vi "Nonlinear Calibration Test v3.vi"() -> ()   [LabVIEW 2009]
doc: "This example illustrates the use of a calibration grid to calibrate and correct an image for nonlinear distortion and accurate shape measurements.\n\nThis example loads the image of a calibration grid used to calibrate the system, learns the grid, then loads an image of parts acquired using the same setup. The example then corrects the image in two ways. The first method corrects the entire image and then measures the area of the coins. The second method corrects only the area of the coins and displays the difference in processing time."
uses:
  <vilib>/vision/NI_Vision_Development_Module.lvlib
panel:
  out "Bottom Image":T1(plugin-control) caption="Coins Image"
  out "Top Image":T1(plugin-control) caption="Calibration Template"
  out "time (ms) to correct":u32
  out "time (ms) to correct":u32
  in  "Load Image of Parts":bool
  in  "Return":bool
  in  "Measure Parts":bool
  in  "Learn Calibration":bool
  in  "Load Calibration Template":bool
  # "1. Loads the image of a calibration grid that is used to calibrate the system."
  # "2. Learn the calibration grid. Note that this process is computation intensive and needs a fair amount of time to complete."
  # "3. Load Image of Parts acquired using the same setup."
  # "4. Correct the image and measure areas of the objects in the image."
  # "This step takes measurements in two ways.  The first calculation corrects \nthe entire image, and then takes the measurements.  The second calculation only corrects the coins, and then takes the measurements."
  # "time (ms) to correct entire image, threshold and calculate measurements"
  # "time (ms) to threshold, correct just coins, and then take measurements"
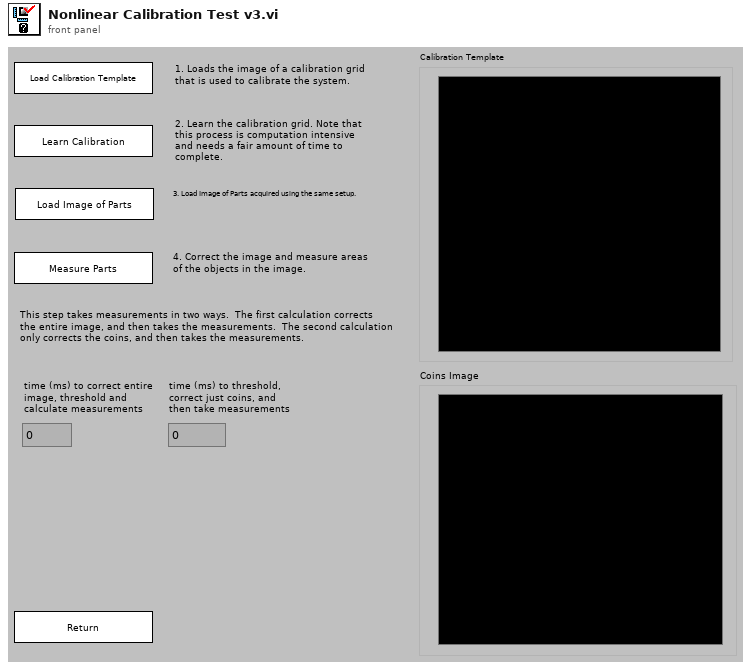
[diagram p1: front panel]
types:
  T1 = typedef "IMAQ Image.ctl" = refnum<image>
  T2 = cluster{"X Step":sgl, "Y Step":sgl, "Unit":u32, "Threshold Range":cluster{"Lower value":sgl, "Upper value":sgl}}
  T3 = cluster{"Distortion":u32, "Corrected Image Scaling":u32, "Corrected Image Learn ROI":u32, "Learn Error Map?":bool, "Learn Correction Table?":bool}
  T4 = typedef "Particle Parameters" = i32
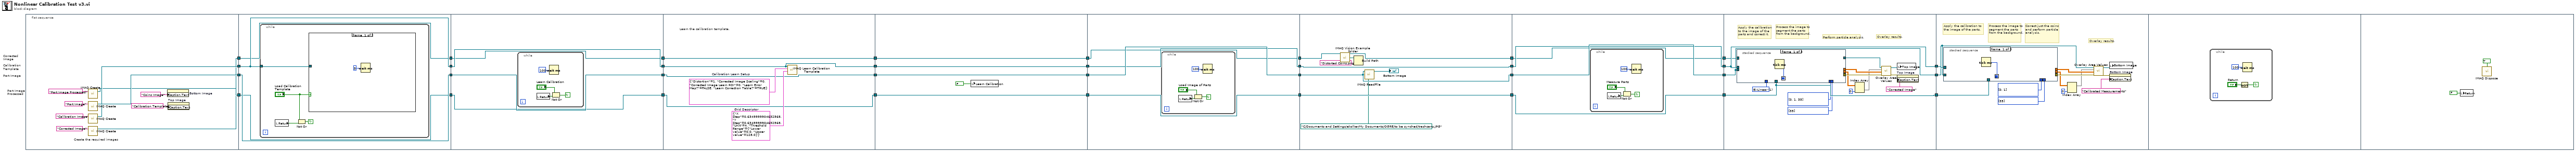
[diagram p0: block diagram]
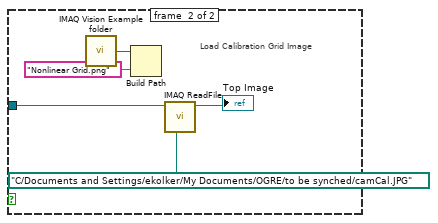
[diagram p2: hidden frame]
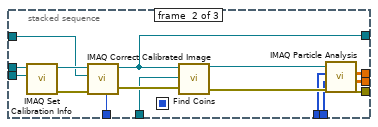
[diagram p3: hidden frame]
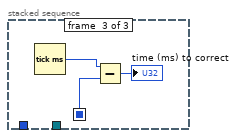
[diagram p4: hidden frame]
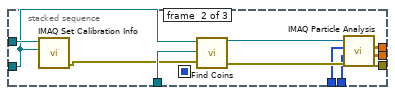
[diagram p5: hidden frame]
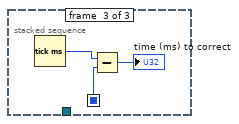
[diagram p6: hidden frame]
diagram:
  # "Corrected\nImage"
  # "Part Image Processed"
  # "Calibration Template"
  # "Part Image"
  n1 = flat-sequence {
    tunnel: [w44] -> w35
    tunnel: [w42] -> w34
    tunnel: [w40] -> w33
    tunnel: [w38] -> w32
    tunnel: w35 -> [w48]
    tunnel: [w48] -> w31
    tunnel: w34 -> [w49]
    tunnel: [w49] -> w30
    tunnel: w33 -> [w47]
    tunnel: [w47] -> w29
    tunnel: w32 -> [w46]
    tunnel: [w46] -> w28
    tunnel: w31 -> [w63]
    tunnel: [w63] -> w27
    tunnel: w30 -> [w62]
    tunnel: [w62] -> w26
    tunnel: w29 -> [w61]
    tunnel: [w61] -> w25
    tunnel: w28 -> [w60]
    tunnel: [w60] -> w24
    tunnel: w27 -> [w70]
    tunnel: [w70] -> w23
    tunnel: w26 -> [w73]
    tunnel: [w73] -> w22
    tunnel: w25 -> [w69]
    tunnel: [w69] -> w21
    tunnel: w24 -> [w68]
    tunnel: [w68] -> w20
    tunnel: w23 -> [w77]
    tunnel: [w77] -> w19
    tunnel: w22 -> [w76]
    tunnel: [w76] -> w18
    tunnel: w21 -> [w75]
    tunnel: [w75] -> w17
    tunnel: w20 -> [w74]
    tunnel: [w74] -> w16
    tunnel: w19 -> [w82]
    tunnel: [w82] -> w15
    tunnel: w18 -> [w81]
    tunnel: [w81] -> w14
    tunnel: w17 -> [w80]
    tunnel: [w80] -> w13
    tunnel: w16 -> [w79]
    tunnel: [w79] -> w12
    tunnel: w15 -> [w94]
    tunnel: [w94] -> w11
    tunnel: w14 -> [w90]
    tunnel: [w90] -> w10
    tunnel: w13 -> [w89]
    tunnel: [w89] -> w9
    tunnel: w12 -> [w88]
    tunnel: [w88] -> w8
    tunnel: w11 -> [w98]
    tunnel: [w98] -> w7
    tunnel: w10 -> [w97]
    tunnel: [w97] -> w6
    tunnel: w9 -> [w96]
    tunnel: [w96] -> w5
    tunnel: w8 -> [w95]
    tunnel: [w95] -> w4
    tunnel: w7 -> [w117]
    tunnel: [w117] -> w3
    tunnel: w6 -> [w118]
    tunnel: [w118] -> w2
    tunnel: w5 -> [w116]
    tunnel: [w116] -> w1
    tunnel: w4 -> [w114]
    tunnel: w3 -> [w144]
    tunnel: w2 -> [w151]
    tunnel: w1 -> [w150]
    frame #0 {
      # "Create the required images"
      n2 = call "IMAQ Create"("Image Name"="Calibration Image") -> ("New Image"=w42:T1)  [unwired: 3 in, 2 out]
      n3 = call "IMAQ Create"("Image Name"="Corrected Image") -> ("New Image"=w38:T1)  [unwired: 3 in, 2 out]
      n4 = call "IMAQ Create"("Image Name"="Part Image Processed") -> ("New Image"=w40:T1)  [unwired: 3 in, 2 out]
      n5 = call "IMAQ Create"("Image Name"="Part Image") -> ("New Image"=w44:T1)  [unwired: 3 in, 2 out]
      n6 = property on="Bottom Image" class="ImageControl"("Caption.Text"="Coins Image" ("Title")) -> ()  [unwired: 2 in, 2 out]
      n7 = property on="Top Image" class="ImageControl"("Caption.Text"="Calibration Template" ("Title")) -> ()  [unwired: 2 in, 2 out]
    }
    frame #1 {
      n8 = while {
        tunnel: w49 -> [w53]
        stop <- w51 continue-if-true
        n9 = local read "Return"() -> (w50:bool)
        n10 = Not Or(1:w50, 2:"Load Calibration Template") -> (0:w51:bool)
        n11 = case shown="True" "Load Calibration Template" {
          tunnel: w53 -> [_ w59]
          frame #0 {
            n12 = Wait (ms)(milliseconds to wait=u32 5) -> ()  [unwired: 1 out]
          }
          frame #1 {
            # "Load Calibration Grid Image"
            n13 = call "IMAQ Vision Example folder.vi"() -> ("Example Image Path"=w58:path)  [unwired: 1 out]
            n14 = Build Path(base path=w58, name or relative path="Nonlinear Grid.png") -> ()  [unwired: 1 out]
            n15 = call "IMAQ ReadFile"("File Path"=path "C:/Documents and Settings/ekolker/My Documents/OGRE/to be synched/camCal.JPG", "Image"=w59) -> ("Image Out"=→"Top Image":T1)  [unwired: 3 in, 6 out]
          }
        }
      }
    }
    frame #2 {
      # "Wait for Learn Calibration Button press"
      n16 = while {
        stop <- w65 continue-if-true
        n17 = local read "Return"() -> (w66:bool)
        n18 = Wait (ms)(milliseconds to wait=u32 100) -> ()  [unwired: 1 out]
        n19 = Not Or(1:w66, 2:"Learn Calibration") -> (0:w65:bool)
      }
    }
    frame #3 {
      w71 = T2 {"X Step"=0.635, "Y Step"=0.635, "Unit"=4, "Threshold Range"={"Lower value"=0.0, "Upper value"=128.0}}  # Grid Descriptor
      w72 = T3 {"Distortion"=1, "Corrected Image Scaling"=0, "Corrected Image Learn ROI"=0, "Learn Error Map?"=FALSE, "Learn Correction Table?"=TRUE}  # Calibration Learn Setup
      # "Learn the calibration template."
      n20 = call "IMAQ Learn Calibration Template"("Grid Descriptor"=w71, "Calibration Learn Setup"=w72, "Image"=w73) -> ()  [unwired: 4 in, 5 out]
    }
    frame #4 {
      n21 = local write "Learn Calibration"(FALSE ("Learn Calibration")) -> ()
    }
    frame #5 {
      n22 = while {
        stop <- w84 continue-if-true
        n23 = local read "Return"() -> (w85:bool)
        n24 = Not Or(1:w85, 2:"Load Image of Parts") -> (0:w84:bool)
        n25 = Wait (ms)(milliseconds to wait=u32 100) -> ()  [unwired: 1 out]
      }
    }
    frame #6 {
      n26 = call "IMAQ Vision Example folder.vi"() -> ("Example Image Path"=w93:path)  [unwired: 1 out]
      n27 = Build Path(base path=w93, name or relative path="Distorted Coins.png") -> ()  [unwired: 1 out]
      n28 = call "IMAQ ReadFile"("File Path"=path "C:/Documents and Settings/ekolker/My Documents/OGRE/to be synched/trashcans.JPG", "Image"=w94) -> ("Image Out"=→"Bottom Image":T1)  [unwired: 3 in, 6 out]
    }
    frame #7 {
      n29 = while {
        stop <- w99 continue-if-true
        n30 = local read "Return"() -> (w101:bool)
        n31 = Not Or(1:w101, 2:"Measure Parts") -> (0:w99:bool)
        n32 = Wait (ms)(milliseconds to wait=u32 100) -> ()  [unwired: 1 out]
      }
    }
    frame #8 {
      w106 = u32 1 items=["Zero Order", "Bi-Linear", "Quadratic", "Cubic Spline"] ("Interpolation Type")
      w113 = T4[] [0, 1, 35] items=["Center of Mass X", "Center of Mass Y", "First Pixel X", "First Pixel Y", "Bounding Rect Left", "Bounding Rect Top", "Bounding Rect Right", "Bounding Rect Bottom", "Max Feret Diameter Start X", "Max Feret Diameter Start Y", "Max Feret Diameter End X", "Max Feret Diameter End Y", "Max Horiz. Segment Length Left", "Max Horiz. Segment Length Right", "Max Horiz. Segment Length Row", "-", "Bounding Rect Width", "Bounding Rect Height", "Bounding Rect Diagonal", "Perimeter", "Convex Hull Perimeter", "Holes' Perimeter", "Max Feret Diameter", "Equivalent Ellipse Major Axis", "Equivalent Ellipse Minor Axis", "Equivalent Ellipse Minor Axis (Feret)", "Equivalent Rect Long Side", "Equivalent Rect Short Side", "Equivalent Rect Diagonal", "Equivalent Rect Short Side (Feret)", "Average Horiz. Segment Length", "Average Vert. Segment Length", "Hydraulic Radius", "Waddel Disk Diameter", "-", "Area", "Holes' Area", "Particle & Holes' Area", "Convex Hull Area", "Image Area", "-", "Number of Holes", "Number of Horiz. Segments", "Number of Vert. Segments", "-", "Orientation", "Max Feret Diameter Orientation", "-", "% Area/Image Area", "% Area/(Particle & Holes' Area)", "Ratio of Equivalent Ellipse Axes", "Ratio of Equivalent Rect Sides", "-", "Elongation Factor", "Compactness Factor", "Heywood Circularity Factor", "Type Factor", "-", "Sum X", "Sum Y", "Sum XX", "Sum XY", "Sum YY", "Sum XXX", "Sum XXY", "Sum XYY", "Sum YYY", "-", "Moment of Inertia XX", "Moment of Inertia XY", "Moment of Inertia YY", "Moment of Inertia XXX", "Moment of Inertia XXY", "Moment of Inertia XYY", "Moment of Inertia YYY", "Norm. Moment of Inertia XX", "Norm. Moment of Inertia XY", "Norm. Moment of Inertia YY", "Norm. Moment of Inertia XXX", "Norm. Moment of Inertia XXY", "Norm. Moment of Inertia XYY", "Norm. Moment of Inertia YYY", "Hu Moment 1", "Hu Moment 2", "Hu Moment 3", "Hu Moment 4", "Hu Moment 5", "Hu Moment 6", "Hu Moment 7"] ("Calibrated Measurements")
      w112 = T4[] [35] items=["Center of Mass X", "Center of Mass Y", "First Pixel X", "First Pixel Y", "Bounding Rect Left", "Bounding Rect Top", "Bounding Rect Right", "Bounding Rect Bottom", "Max Feret Diameter Start X", "Max Feret Diameter Start Y", "Max Feret Diameter End X", "Max Feret Diameter End Y", "Max Horiz. Segment Length Left", "Max Horiz. Segment Length Right", "Max Horiz. Segment Length Row", "-", "Bounding Rect Width", "Bounding Rect Height", "Bounding Rect Diagonal", "Perimeter", "Convex Hull Perimeter", "Holes' Perimeter", "Max Feret Diameter", "Equivalent Ellipse Major Axis", "Equivalent Ellipse Minor Axis", "Equivalent Ellipse Minor Axis (Feret)", "Equivalent Rect Long Side", "Equivalent Rect Short Side", "Equivalent Rect Diagonal", "Equivalent Rect Short Side (Feret)", "Average Horiz. Segment Length", "Average Vert. Segment Length", "Hydraulic Radius", "Waddel Disk Diameter", "-", "Area", "Holes' Area", "Particle & Holes' Area", "Convex Hull Area", "Image Area", "-", "Number of Holes", "Number of Horiz. Segments", "Number of Vert. Segments", "-", "Orientation", "Max Feret Diameter Orientation", "-", "% Area/Image Area", "% Area/(Particle & Holes' Area)", "Ratio of Equivalent Ellipse Axes", "Ratio of Equivalent Rect Sides", "-", "Elongation Factor", "Compactness Factor", "Heywood Circularity Factor", "Type Factor", "-", "Sum X", "Sum Y", "Sum XX", "Sum XY", "Sum YY", "Sum XXX", "Sum XXY", "Sum XYY", "Sum YYY", "-", "Moment of Inertia XX", "Moment of Inertia XY", "Moment of Inertia YY", "Moment of Inertia XXX", "Moment of Inertia XXY", "Moment of Inertia XYY", "Moment of Inertia YYY", "Norm. Moment of Inertia XX", "Norm. Moment of Inertia XY", "Norm. Moment of Inertia YY", "Norm. Moment of Inertia XXX", "Norm. Moment of Inertia XXY", "Norm. Moment of Inertia XYY", "Norm. Moment of Inertia YYY", "Hu Moment 1", "Hu Moment 2", "Hu Moment 3", "Hu Moment 4", "Hu Moment 5", "Hu Moment 6", "Hu Moment 7"] ("Pixel Measurements")
      # "Overlay results."
      # "Perform particle analysis."
      # "Process the image to segment the parts from the background."
      # "Apply the calibration to the image of the parts and correct it."
      n33 = stacked-sequence {
        seq-local: [w119 _ _] -> [_ _ w137]
        tunnel: w118 -> [_ w134 _]
        tunnel: w117 -> [_ w133 _]
        tunnel: w116 -> [_ w130 _]
        tunnel: [_ w128 _] -> w115
        tunnel: w114 -> [_ w127 _]
        tunnel: w113 -> [_ w125 _]
        tunnel: w112 -> [_ w124 _]
        tunnel: [_ w123 _] -> w111
        tunnel: [_ w122 _] -> w109
        tunnel: [_ w121 _] -> w107
        tunnel: w106 -> [_ w120 _]
        frame #0 {
          n34 = Tick Count (ms)() -> (millisecond timer value=w119:u32)
        }
        frame #1 {
          n35 = call "IMAQ Set Calibration Info"("Image Dst"=w133, "Image Src"=w134) -> ("error out"=w132:errorcluster, "Calibrated Image"=w135:T1)  [unwired: 2 in, 6 out]
          n36 = call "IMAQ Correct Calibrated Image"("Interpolation Type"=w120, "error in (no error)"=w132, "Image Dst"=w127, "Image Src"=w135) -> ("error out"=w131:errorcluster, "Corrected Image"=w121:T1)  [unwired: 3 in, 3 out]
          n37 = call "Find Coins.vi"("error in"=w131, "Dest Image"=w130, "Source Image"=w121) -> ("error out"=w129:errorcluster, "Image Out"=w126:T1)  [unwired: 1 out]
          n38 = call "IMAQ Particle Analysis"("error in (no error)"=w129, "Real-World Measurements"=w124, "Pixel Measurements"=w125, "Image"=w126) -> ("error out"=w128:errorcluster, "Particle Measurements (Real-World)"=w122:dbl[][], "Particle Measurements (Pixels)"=w123:dbl[][])  [unwired: 1 in, 4 out]
        }
        frame #2 {
          n39 = Tick Count (ms)() -> (millisecond timer value=w138:u32)
          n40 = Subtract(x=w138, y=w137) -> (x-y=→"time (ms) to correct":u32)
        }
      }
      n41 = Index Array(array=w109, index (col)=0 ("Index (row)")) -> (element=w110:dbl[])  [unwired: 1 in]
      n42 = call "Overlay Area Values.vi"("error in (no error)"=w115, "Coin Center (X,Y)"=w111, "Measurement Values"=w110, "Image In"=w107) -> ("error out"=w104:errorcluster, "Image Out"=w105:T1)  [unwired: 2 out]
      n43 = local write "Top Image"(w105) -> ()
      n44 = property on="Top Image" class="ImageControl"(error in=w104, "Caption.Text"="Corrected Image" ("Title")) -> ()  [unwired: 1 in, 2 out]
    }
    frame #9 {
      w143 = T4[] [0, 1] items=["Center of Mass X", "Center of Mass Y", "First Pixel X", "First Pixel Y", "Bounding Rect Left", "Bounding Rect Top", "Bounding Rect Right", "Bounding Rect Bottom", "Max Feret Diameter Start X", "Max Feret Diameter Start Y", "Max Feret Diameter End X", "Max Feret Diameter End Y", "Max Horiz. Segment Length Left", "Max Horiz. Segment Length Right", "Max Horiz. Segment Length Row", "-", "Bounding Rect Width", "Bounding Rect Height", "Bounding Rect Diagonal", "Perimeter", "Convex Hull Perimeter", "Holes' Perimeter", "Max Feret Diameter", "Equivalent Ellipse Major Axis", "Equivalent Ellipse Minor Axis", "Equivalent Ellipse Minor Axis (Feret)", "Equivalent Rect Long Side", "Equivalent Rect Short Side", "Equivalent Rect Diagonal", "Equivalent Rect Short Side (Feret)", "Average Horiz. Segment Length", "Average Vert. Segment Length", "Hydraulic Radius", "Waddel Disk Diameter", "-", "Area", "Holes' Area", "Particle & Holes' Area", "Convex Hull Area", "Image Area", "-", "Number of Holes", "Number of Horiz. Segments", "Number of Vert. Segments", "-", "Orientation", "Max Feret Diameter Orientation", "-", "% Area/Image Area", "% Area/(Particle & Holes' Area)", "Ratio of Equivalent Ellipse Axes", "Ratio of Equivalent Rect Sides", "-", "Elongation Factor", "Compactness Factor", "Heywood Circularity Factor", "Type Factor", "-", "Sum X", "Sum Y", "Sum XX", "Sum XY", "Sum YY", "Sum XXX", "Sum XXY", "Sum XYY", "Sum YYY", "-", "Moment of Inertia XX", "Moment of Inertia XY", "Moment of Inertia YY", "Moment of Inertia XXX", "Moment of Inertia XXY", "Moment of Inertia XYY", "Moment of Inertia YYY", "Norm. Moment of Inertia XX", "Norm. Moment of Inertia XY", "Norm. Moment of Inertia YY", "Norm. Moment of Inertia XXX", "Norm. Moment of Inertia XXY", "Norm. Moment of Inertia XYY", "Norm. Moment of Inertia YYY", "Hu Moment 1", "Hu Moment 2", "Hu Moment 3", "Hu Moment 4", "Hu Moment 5", "Hu Moment 6", "Hu Moment 7"] ("Calibrated Measurements")
      w148 = T4[] [35] items=["Center of Mass X", "Center of Mass Y", "First Pixel X", "First Pixel Y", "Bounding Rect Left", "Bounding Rect Top", "Bounding Rect Right", "Bounding Rect Bottom", "Max Feret Diameter Start X", "Max Feret Diameter Start Y", "Max Feret Diameter End X", "Max Feret Diameter End Y", "Max Horiz. Segment Length Left", "Max Horiz. Segment Length Right", "Max Horiz. Segment Length Row", "-", "Bounding Rect Width", "Bounding Rect Height", "Bounding Rect Diagonal", "Perimeter", "Convex Hull Perimeter", "Holes' Perimeter", "Max Feret Diameter", "Equivalent Ellipse Major Axis", "Equivalent Ellipse Minor Axis", "Equivalent Ellipse Minor Axis (Feret)", "Equivalent Rect Long Side", "Equivalent Rect Short Side", "Equivalent Rect Diagonal", "Equivalent Rect Short Side (Feret)", "Average Horiz. Segment Length", "Average Vert. Segment Length", "Hydraulic Radius", "Waddel Disk Diameter", "-", "Area", "Holes' Area", "Particle & Holes' Area", "Convex Hull Area", "Image Area", "-", "Number of Holes", "Number of Horiz. Segments", "Number of Vert. Segments", "-", "Orientation", "Max Feret Diameter Orientation", "-", "% Area/Image Area", "% Area/(Particle & Holes' Area)", "Ratio of Equivalent Ellipse Axes", "Ratio of Equivalent Rect Sides", "-", "Elongation Factor", "Compactness Factor", "Heywood Circularity Factor", "Type Factor", "-", "Sum X", "Sum Y", "Sum XX", "Sum XY", "Sum YY", "Sum XXX", "Sum XXY", "Sum XYY", "Sum YYY", "-", "Moment of Inertia XX", "Moment of Inertia XY", "Moment of Inertia YY", "Moment of Inertia XXX", "Moment of Inertia XXY", "Moment of Inertia XYY", "Moment of Inertia YYY", "Norm. Moment of Inertia XX", "Norm. Moment of Inertia XY", "Norm. Moment of Inertia YY", "Norm. Moment of Inertia XXX", "Norm. Moment of Inertia XXY", "Norm. Moment of Inertia XYY", "Norm. Moment of Inertia YYY", "Hu Moment 1", "Hu Moment 2", "Hu Moment 3", "Hu Moment 4", "Hu Moment 5", "Hu Moment 6", "Hu Moment 7"] ("Pixel Measurements")
      # "Overlay results."
      # "Correct just the coins and perform particle analysis."
      # "Process the image to segment the parts from the background."
      # "Apply the calibration to the image of the parts."
      n45 = stacked-sequence {
        seq-local: [w152 _ _] -> [_ _ w165]
        tunnel: w151 -> [_ w163 _]
        tunnel: w150 -> [_ w162 _]
        tunnel: [_ w160 _] -> w149
        tunnel: w148 -> [_ w153 _]
        tunnel: [_ w158 _] -> w147
        tunnel: [_ w157 _] -> w146
        tunnel: w144 -> [_ w156 _]
        tunnel: w143 -> [_ w154 _]
        frame #0 {
          n46 = Tick Count (ms)() -> (millisecond timer value=w152:u32)
        }
        frame #1 {
          n47 = call "IMAQ Set Calibration Info"("Image Dst"=w156, "Image Src"=w163) -> ("error out"=w155:errorcluster)  [unwired: 2 in, 7 out]
          n48 = call "Find Coins.vi"("error in"=w155, "Dest Image"=w162, "Source Image"=w156) -> ("error out"=w161:errorcluster, "Image Out"=w159:T1)  [unwired: 1 out]
          n49 = call "IMAQ Particle Analysis"("error in (no error)"=w161, "Real-World Measurements"=w153, "Pixel Measurements"=w154, "Image"=w159) -> ("error out"=w160:errorcluster, "Particle Measurements (Real-World)"=w157:dbl[][], "Particle Measurements (Pixels)"=w158:dbl[][])  [unwired: 1 in, 4 out]
        }
        frame #2 {
          n50 = Tick Count (ms)() -> (millisecond timer value=w166:u32)
          n51 = Subtract(x=w166, y=w165) -> (x-y=→"time (ms) to correct":u32)
        }
      }
      n52 = Index Array(array=w146, index (col)=0 ("Index (row)")) -> (element=w142:dbl[])  [unwired: 1 in]
      n53 = call "Overlay Area Values.vi"("error in (no error)"=w149, "Coin Center (X,Y)"=w147, "Measurement Values"=w142, "Image In"=w144) -> ("error out"=w140:errorcluster, "Image Out"=w141:T1)  [unwired: 2 out]
      n54 = local write "Bottom Image"(w141) -> ()
      n55 = property on="Bottom Image" class="ImageControl"(error in=w140, "Caption.Text"="Calibrated Measurements" ("Title")) -> ()  [unwired: 1 in, 2 out]
    }
    frame #10 {
      n56 = while {
        stop <- w167 continue-if-true
        n57 = Not(x="Return") -> (.not. x?=w167:bool)
        n58 = Wait (ms)(milliseconds to wait=u32 100) -> ()  [unwired: 1 out]
      }
    }
    frame #11 {
      n59 = local write "Return"(FALSE ("Return")) -> ()
      n60 = call "IMAQ Dispose"("All Images? (No)"=TRUE) -> ()  [unwired: 2 in, 4 out]
    }
  }
